vi "CALC_TRAN_COUP_PAR.vi"(0 "VISA IN":refnum<visa-resource-name>, 1 "Parameters to Couple":T1(ring), 5 "error in":errorcluster, 7 "Channel":i32=1) -> (14 "VISA Out":refnum<visa-resource-name>, 19 "error out":errorcluster)   [LabVIEW 2018, in "PNA-X.lvlib"]
doc: "CALCulate<cnum>:TRANsform:COUPle:PARameters <num> \n(Read-Write) Specifies the time domain transform parameters to be coupled. The settings for those \nparameters will be copied from the selected measurement to all other measurements on the channel. \nTo turn coupling ON and OFF, use SENS:COUP:PAR \nTo specify Gating parameters to couple, use CALC:FILT:COUP:PAR \nLearn more about Time Domain Trace Coupling \nSee Critical Note \nParameters \n<cnum> Channel number of the measurement. There must be a selected measurement \non that channel. If unspecified, <cnum> is set to 1. \n<num> (Numeric) Parameters to couple. To specify more than one parameter, add the \n1566\n\nnumbers. \n1 - Transform Stimulus (Start, Stop, Center, and Span TIME settings.) \n2 - Transform State (ON / OFF) \n4 - Transform Window (Kaiser Beta / Impulse Width) \n8 - Transform Mode (Low Pass Impulse, Low Pass Step, Band Pass) \n16 - Transform Distance Marker Units \nExamples 'To couple all parameters: \nCALC:TRAN:COUP:PAR 31 \n'To couple Stimulus and Mode: \ncalculate2:transform:couple:parameters 9 \nQuery Syntax CALCulate<cnum>:TRANsform:COUPle:PARameters? \nReturn Type Numeric \nDefault 29 (All parameters except 2 - Transform State)"
uses:
  PNA-X.lvlib
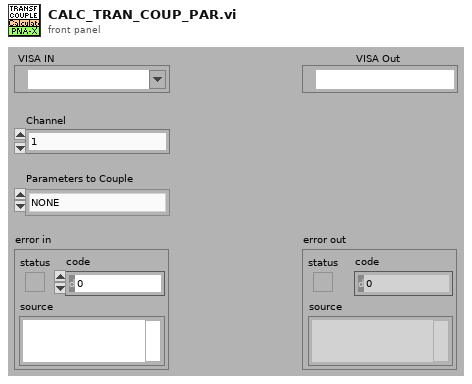
[diagram p1: front panel]
types:
  T1 = enum16{"NONE", "Stimulus", "State (ON/OFF)", "Stimulus, State", "Window (Kaiser Bets / Impulse Width)", "Window, Stimulus", "Window, State", "Window, State, Stimulus", "Mode (Low Pass Impulse, Low Pass Step, Band Pass)", "Mode, Stimulus", "Mode, State", "Mode, State, Stimulus", "Mode, Window", "Mode, Window, Stimulus", "Mode, Window, State", "Mode, Window, State, Stimulus", "Distance Marker Units", "Distance, Stimulus", "Distance, State", "Distance, State, Stimulus", "Distance, Window", "Distance, Window, Stimulus", "Distance, Window, State", "Distance, Window, State, Stimulus", "Distance, Mode", "Distance, Mode, Stimulus", "Distance, Mode, State", "Distance, Mode, State, Stimulus", "Distance, Mode, Window", "Distance, Mode, Window, Stimulus", "Distance, Mode, Window, State", "Distance, Mode, Window, State, Stimulus"}
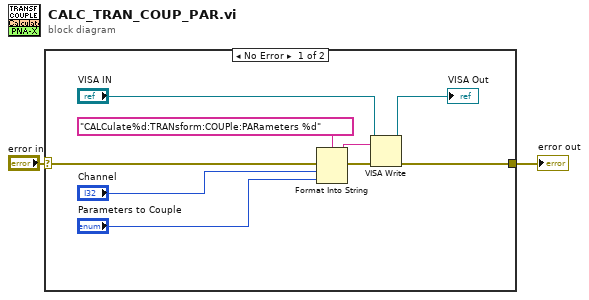
[diagram p0: block diagram]
diagram:
  n1 = case shown="No Error" "error in" {
    selector: "error in" -> [w11 w12]
    tunnel: [w6 w12] -> w1
    frame No Error {
      n2 = Format Into String(format string="CALCulate%d:TRANsform:COUPle:PARameters %d" ("Cmdline"), error in=w11, "Channel", "Parameters to Couple") -> (resulting string=w9:string, error out=w10:errorcluster)  [unwired: 1 in]
      n3 = VISA Write(VISA resource name="VISA IN", write buffer=w9, error in (no error)=w10) -> (VISA resource name out=→"VISA Out":refnum<visa-resource-name>, error out=w6:errorcluster)  [unwired: 1 out]
    }
    frame Error {
    }
  }
  "error out" <- w1
